vi "Compass PD test.vi"() -> ()   [LabVIEW 2012]
uses:
  <vilib>/robotics/Controls/Compass Indicator/Compass Indicator.xctl
  <vilib>/Platform/TimedLoop/XDataNode/timing_clust.ctl
  <vilib>/Platform/TimedLoop/XDataNode/nitl_modes.ctl
  <vilib>/Platform/TimedLoop/XDataNode/wakeup.ctl
  <vilib>/Analysis/coordinate.llb/Angle Units.ctl
  <vilib>/Analysis/coordinate.llb/Angle Range (Degree).ctl
  <vilib>/Analysis/coordinate.llb/Wrap Angle (scalar).vi
  <vilib>/platform/TimedLoop/XDataNode/XDataNode.xnode
  <vilib>/Analysis/NI_AAL_Angle.lvlib
  <vilib>/Platform/TimedLoop/XDataNode/XDNodeRunTimeDep.lvlib
panel:
  in  "Ki":dbl
  in  "Kd":dbl=0.2
  in  "Kp":dbl=0.2
  in  "Slide":dbl(slide) min=0.0 max=360.0 step=0.1 scale=0.0..360.0
  out "Compass Indicator":dbl(xcontrol)
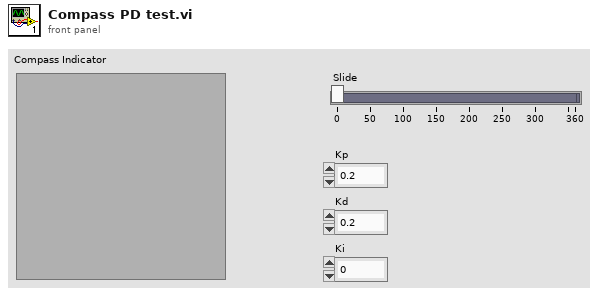
[diagram p1: front panel]
types:
  T1 = typedef "XDNodeRunTimeDep.lvlib/timing_clust.ctl" = cluster{"Expected End [f-1]":u64, "Actual End [f-1]":u64, "Finished Late? [f-1]":bool, "Expected End [i-1]":u64, "Actual End [i-1]":u64, "Finished Late? [i-1]":bool, "Expected Start [i]":u64, "Actual Start [i]":u64, "Expected Start [f]":u64, "Actual Start [f]":u64, "Source Name":string, "Structure Name":string, "Period":i64, "Deadline":i64, "Offset":i64, "Start":i64, "Priority":i32, "Timeout":i32, "Mode":T2, "Wakeup Reason":T3, "Error":errorcluster, "Source Type":string, "Secondary Source Type":string, "Global End Time":u64, "Global Start Time":u64, "Frame Duration":u64, "Iteration Duration":u64, "Assigned CPU":i32, "I/O Scan Engine Mode":u32}
  T2 = typedef "XDNodeRunTimeDep.lvlib/nitl_modes.ctl" = enum32{"No Change", "Process missed periods, maintain original phase", "Discard missed periods, maintain original phase", "Process missed periods, ignore original phase", "Discard missed periods, ignore original phase"}
  T3 = typedef "XDNodeRunTimeDep.lvlib/wakeup.ctl" = enum32{"Normal", "Aborted", "Asynchronous wakeup", "Timing source error", "Timed loop error", "Timeout"}
  T4 = typedef "NI_AAL_Angle.lvlib/Angle Range (Degree).ctl" = u16
  T5 = typedef "NI_AAL_Angle.lvlib/Angle Units.ctl" = i32
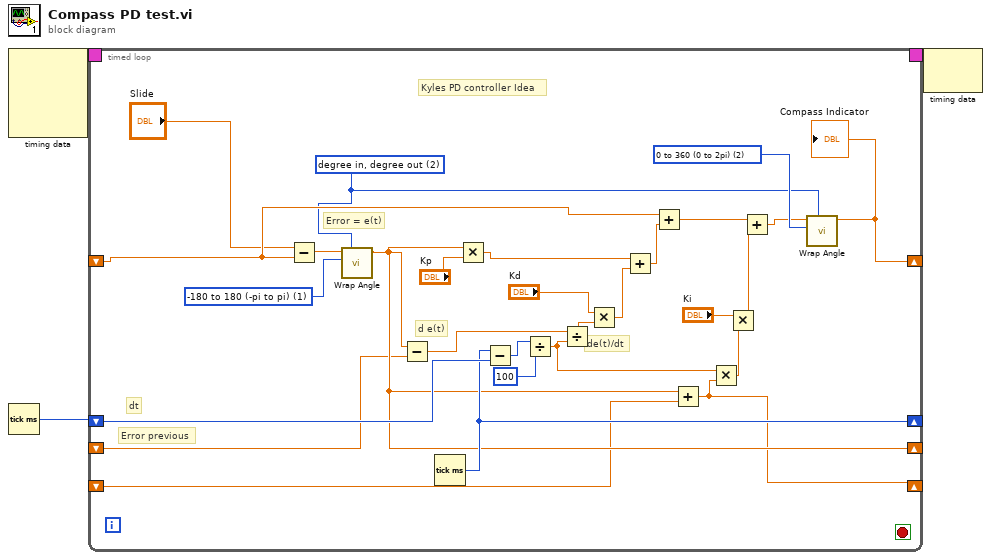
[diagram p0: block diagram]
diagram:
  n1 = node-c288() -> (w3:T1)  [unwired: 4 in]
  n2 = Tick Count (ms)() -> (millisecond timer value=w1:u32)
  n3 = timed-loop {
    timing: w3 -> [_]
    timing-out: [_] -> w2
    shift-right: [w12] -> _
    shift-left: _ -> [w11]
    shift-right: [w24] -> _
    shift-left: w1 -> [w25]
    shift-right: [w20] -> _
    shift-left: _ -> [w21]
    shift-right: [w8] -> _
    shift-left: _ -> [w10]
    stop <- _ stop-if-true
    w16 = T4 1 items=["none", "-180 to 180 (-pi to pi)", "0 to 360 (0 to 2pi)"] ("angle range")
    w19 = T4 2 items=["none", "-180 to 180 (-pi to pi)", "0 to 360 (0 to 2pi)"] ("angle range")
    w17 = T5 2 items=["radian in, radian out", "radian in, degree out", "degree in, degree out", "degree in, radian out"] ("angle units")
    # "Error previous"
    # "dt"
    # "d e(t)"
    # "de(t)/dt"
    # "Error = e(t)"
    # "Kyles PD controller Idea"
    n4 = Subtract(x="Slide", y=w21) -> (x-y=w18:dbl)
    n5 = call-poly <vilib>:"Wrap Angle.vi"("angle units"=w17, "angle range"=w16, "angle in"=w18) -> ("angle out"=w12:dbl)  [unwired: 7 in, 1 out]
    n6 = Subtract(x=w12, y=w11) -> (x-y=w30:dbl)
    n7 = Tick Count (ms)() -> (millisecond timer value=w24:u32)
    n8 = Multiply(x=w12, y="Kp") -> (x*y=w15:dbl)
    n9 = Subtract(x=w24, y=w25) -> (x-y=w29:u32)
    n10 = Divide(x=w29, y=u32 100) -> (x/y=w9:dbl)
    n11 = Divide(x=w30, y=w9) -> (x/y=w28:dbl)
    n12 = Multiply(x="Kd", y=w28) -> (x*y=w26:dbl)
    n13 = Add(x=w15, y=w26) -> (x+y=w14:dbl)
    n14 = Add(x=w21, y=w14) -> (x+y=w22:dbl)
    n15 = Add(x=w12, y=w10) -> (x+y=w8:dbl)
    n16 = Multiply(x=w9, y=w8) -> (x*y=w6:dbl)
    n17 = Multiply(x="Ki", y=w6) -> (x*y=w5:dbl)
    n18 = Add(x=w22, y=w5) -> (x+y=w7:dbl)
    n19 = call-poly <vilib>:"Wrap Angle.vi"("angle units"=w17, "angle range"=w19, "angle in"=w7) -> ("angle out"=w20:dbl)  [unwired: 7 in, 1 out]
    "Compass Indicator" <- w20
  }
  n20 = node-c288(w2) -> ()  [unwired: 1 out]
